vi "Logger.FindData2.vi"() -> ()   [LabVIEW 2016]
uses:
  Logger.File.Serials.ctl
  Sequence/Sequence.Step.Status.ctl
panel:
  out "spreadsheet string 2":string
  out "spreadsheet string":string
  out "Array":string[](array[string])
  out "unique values":string[](array[string])
  out "sum":i16
  out "sorted array 2":T1(array[cluster])
  out "Data":T2[][](array[typedef])
  out "error out":errorcluster
  out "size(s)":i32
  in  "Files":path[](array[path])=[path "D:/Maszup/WABCO/SVN/LaserMarkingStation/SOFTWARE/logs/results1/new/170424160700 899 053 814 4.tdms", path "D:/Maszup/WABCO/SVN/LaserMarkingStation/SOFTWARE/logs/results1/new/170425142313 899 053 814 4.tdms", path "D:/Maszup/WABCO/SVN/LaserMarkingStation/SOFTWARE/logs/results1/new/170425154602 899 053 814 4.tdms", path "D:/Maszup/WABCO/SVN/LaserMarkingStation/SOFTWARE/logs/results1/new/170425215851 899 053 814 4.tdms", path "D:/Maszup/WABCO/SVN/LaserMarkingStation/SOFTWARE/logs/results1/new/170427101020 899 053 814 4.tdms", path "D:/Maszup/WABCO/SVN/LaserMarkingStation/SOFTWARE/logs/results1/new/170427132145 899 053 814 4.tdms", path "D:/Maszup/WABCO/SVN/LaserMarkingStation/SOFTWARE/logs/results1/new/170427164857 899 053 814 4.tdms", path "D:/Maszup/WABCO/SVN/LaserMarkingStation/SOFTWARE/logs/results1/old/170404114910 899 053 814 4.tdms", path "D:/Maszup/WABCO/SVN/LaserMarkingStation/SOFTWARE/logs/results1/old/170404165439 899 053 814 4.tdms", path "D:/Maszup/WABCO/SVN/LaserMarkingStation/SOFTWARE/logs/results1/old/170404212337 899 053 814 4.tdms", path "D:/Maszup/WABCO/SVN/LaserMarkingStation/SOFTWARE/logs/results1/old/170406132445 899 053 814 4.tdms", path "D:/Maszup/WABCO/SVN/LaserMarkingStation/SOFTWARE/logs/results1/old/170406155100 899 053 814 4.tdms", path "D:/Maszup/WABCO/SVN/LaserMarkingStation/SOFTWARE/logs/results1/old/170406203614 899 053 814 4.tdms", path "D:/Maszup/WABCO/SVN/LaserMarkingStation/SOFTWARE/logs/results1/old/170408024126 899 053 814 4.tdms", path "D:/Maszup/WABCO/SVN/LaserMarkingStation/SOFTWARE/logs/results1/old/170408025114 899 053 814 4.tdms", path "D:/Maszup/WABCO/SVN/LaserMarkingStation/SOFTWARE/logs/results1/old/170408033252 899 053 814 4.tdms", path "D:/Maszup/WABCO/SVN/LaserMarkingStation/SOFTWARE/logs/results1/old/170410070739 899 053 814 4.tdms", path "D:/Maszup/WABCO/SVN/LaserMarkingStation/SOFTWARE/logs/results1/old/170410115154 899 053 814 4.tdms", path "D:/Maszup/WABCO/SVN/LaserMarkingStation/SOFTWARE/logs/results1/old/170411223457 899 053 814 4.tdms", path "D:/Maszup/WABCO/SVN/LaserMarkingStation/SOFTWARE/logs/results1/old/170412013424 899 053 814 4.tdms", path "D:/Maszup/WABCO/SVN/LaserMarkingStation/SOFTWARE/logs/results1/old/170412052729 899 053 814 4.tdms", path "D:/Maszup/WABCO/SVN/LaserMarkingStation/SOFTWARE/logs/results1/old/170413051815 899 053 814 4.tdms", path "D:/Maszup/WABCO/SVN/LaserMarkingStation/SOFTWARE/logs/results1/old/170413111535 899 053 814 4.tdms", path "D:/Maszup/WABCO/SVN/LaserMarkingStation/SOFTWARE/logs/results1/old/170413172133 899 053 814 4.tdms", path "D:/Maszup/WABCO/SVN/LaserMarkingStation/SOFTWARE/logs/results1/old/170414192304 899 053 814 4.tdms", path "D:/Maszup/WABCO/SVN/LaserMarkingStation/SOFTWARE/logs/results1/old/170419031847 899 053 814 4.tdms", path "D:/Maszup/WABCO/SVN/LaserMarkingStation/SOFTWARE/logs/results1/old/170419071455 899 053 814 4.tdms", path "D:/Maszup/WABCO/SVN/LaserMarkingStation/SOFTWARE/logs/results2/new/170420162556 899 053 814 4.tdms", path "D:/Maszup/WABCO/SVN/LaserMarkingStation/SOFTWARE/logs/results2/new/170421075116 899 053 814 4.tdms", path "D:/Maszup/WABCO/SVN/LaserMarkingStation/SOFTWARE/logs/results2/new/170424124919 899 053 814 4.tdms", path "D:/Maszup/WABCO/SVN/LaserMarkingStation/SOFTWARE/logs/results2/new/170425130831 899 053 814 4.tdms"]
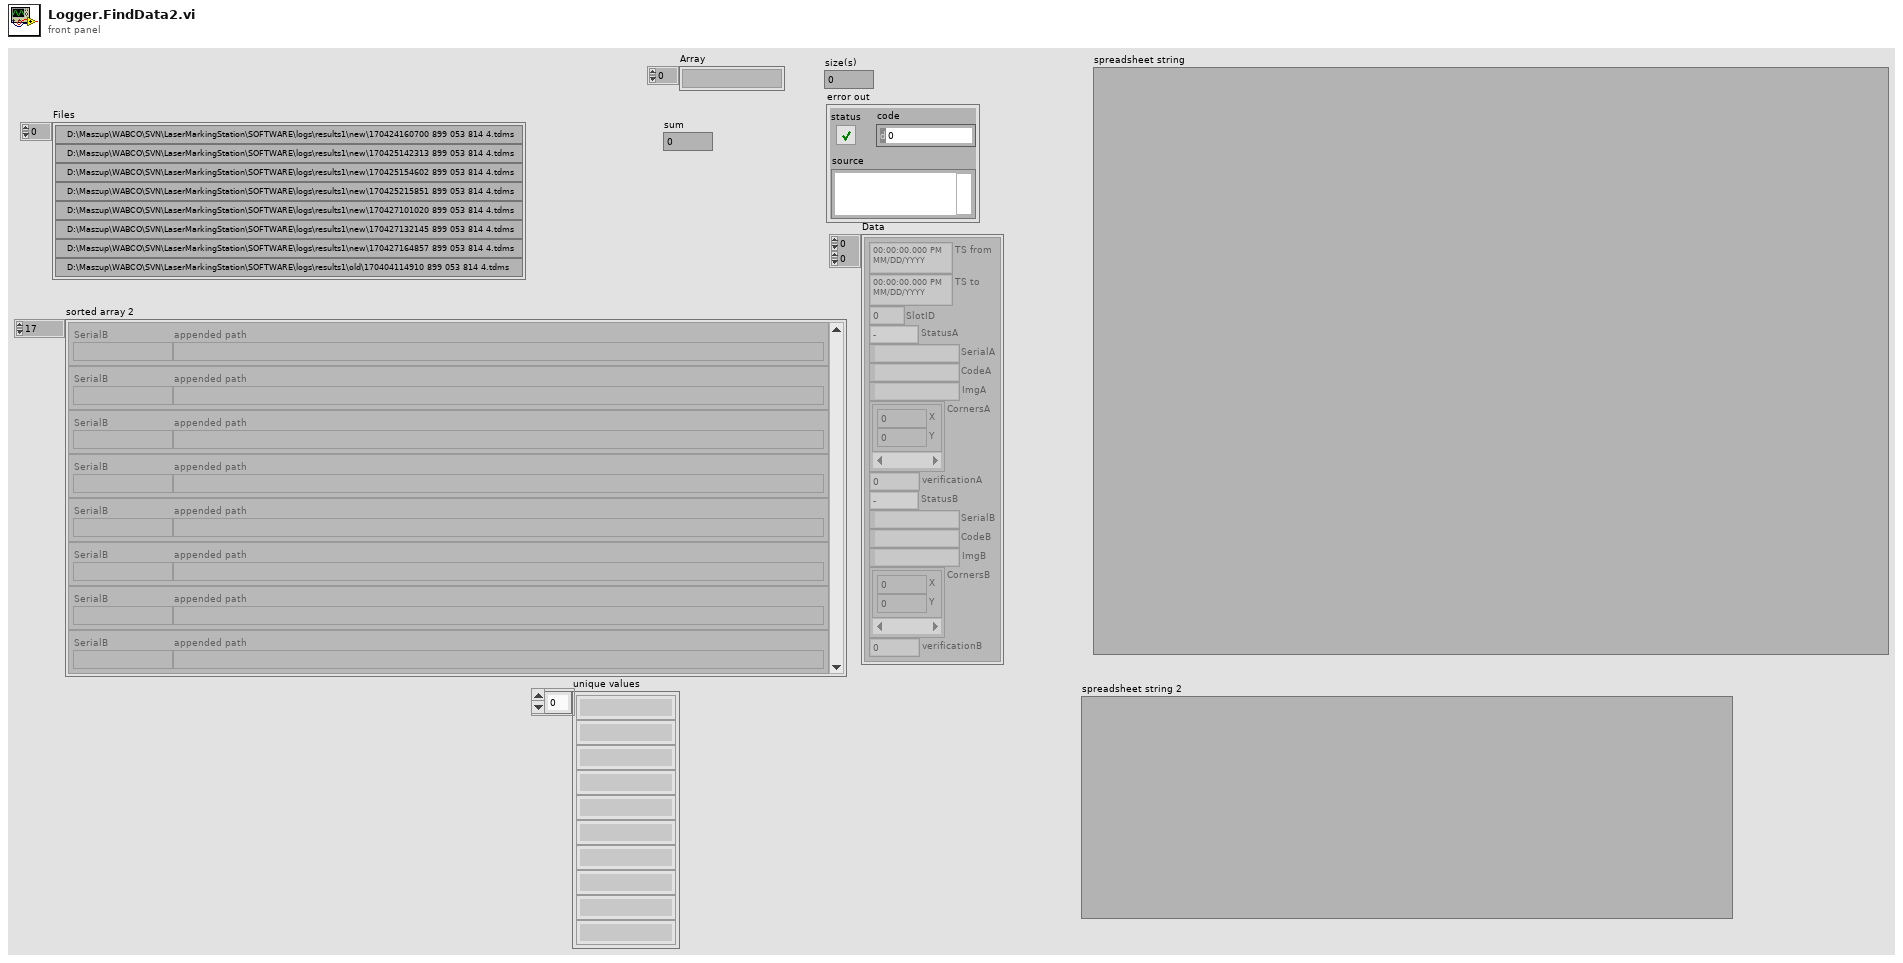
[diagram p1: front panel]
types:
  T1 = cluster{"SerialB":string, "appended path":path}[]
  T2 = typedef "Logger.File.Serials.ctl" = cluster{"TS from":timestamp, "TS to":timestamp, "SlotID":u8, "StatusA":T3, "SerialA":string, "CodeA":string, "ImgA":string, "CornersA":cluster{"X":i32, "Y":i32}[], "verificationA":u8, "StatusB":T3, "SerialB":string, "CodeB":string, "ImgB":string, "CornersB":cluster{"X":i32, "Y":i32}[], "verificationB":u8}
  T3 = typedef "Sequence.Step.Status.ctl" = enum16{"-", "Pending", "Running", "Skipped", "Passed", "Failed", "Done", "Error", "Aborted", "Stopped"}
  T4 = enum16{"open", "open or create", "create or replace", "create", "open (read-only)"}
  T5 = cluster{"SerialB":string, "appended path":path, i32}
  T6 = cluster{"SerialB":string, "appended path":path, i32}[]
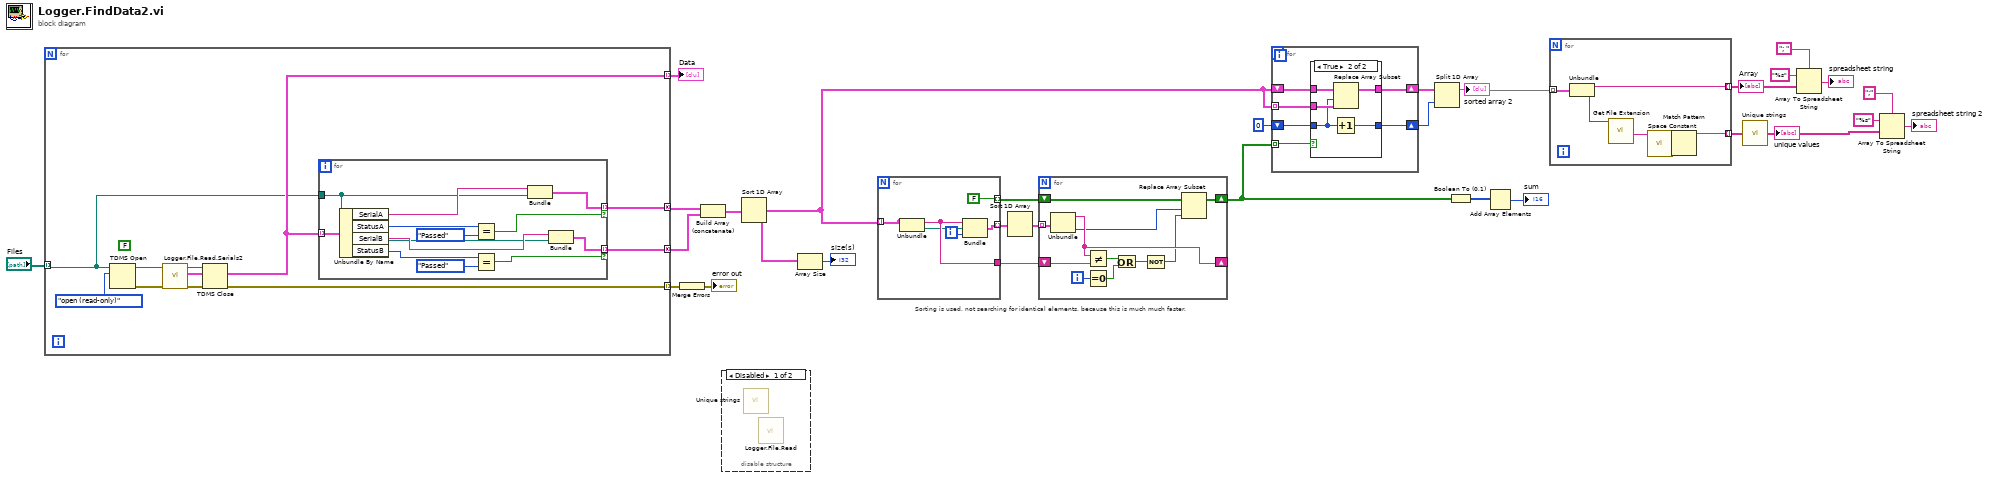
[diagram p0: block diagram]
diagram:
  # "Sorting is used, not searching for identical elements, because this is much much faster."
  n1 = for {
    tunnel: "Files" -> [w30] mode=indexing
    tunnel: [w32] -> w26 mode=indexing
    tunnel: [w39] -> w23 mode=concatenating
    tunnel: [w38] -> w24 mode=concatenating
    tunnel: [w31] -> w22 mode=indexing
    (unwired) FALSE ("create index file? (T)")
    n2 = TDMS Open(10:T4."open (read-only)" ("operation (0:open)"), 11:w30) -> (0:w35:errorcluster, 3:w36:refnum<k34>)  [unwired: 5 in]
    n3 = call "Logger.File.Read.Serials2.vi"("error in"=w35, "file ref in"=w36) -> ("error out"=w34:errorcluster, "Data"=w31:T2[], "file ref out"=w33:refnum<k34>)  [unwired: 7 in]
    n4 = TDMS Close(8:w34, 11:w33) -> (0:w32:errorcluster)  [unwired: 1 out]
    n5 = for {
      tunnel: [w40] -> w39 mode=indexing if=w47
      tunnel: [w41] -> w38 mode=indexing if=w46
      tunnel: w31 -> [w45] mode=indexing
      tunnel: w30 -> [w42]
      n6 = Unbundle By Name(w45) -> ("SerialA"=w44:string, "StatusA"=w51:T3, "SerialB"=w43:string, "StatusB"=w48:T3)
      n7 = Equal?(x=w51, y=Sequence.Step.Status."Passed") -> (x = y?=w46:bool)
      n8 = Equal?(x=w48, y=Sequence.Step.Status."Passed") -> (x = y?=w47:bool)
      n9 = Bundle("SerialA"=w44, "appended path"=w42) -> (w41:cluster{"SerialA":string, "appended path":path})  [unwired: 1 in]
      n10 = Bundle("SerialB"=w43, "appended path"=w42) -> (w40:cluster{"SerialB":string, "appended path":path})  [unwired: 1 in]
    }
  }
  "Data" <- w22
  n11 = Merge Errors(w26) -> (→"error out":errorcluster)
  n12 = Build Array (concatenate)(w24, w23) -> (w28:T1)
  n13 = disable-structure shown="Disabled" {
    frame Disabled {
      n14 = call "Unique strings.vi"() -> ()  [unwired: 1 in, 1 out]
      n15 = call "Logger.File.Read.vi"() -> ()  [unwired: 8 in, 4 out]
    }
    frame Enabled {
    }
  }
  n16 = Sort 1D Array(array=w28) -> (sorted array=w12:T1)
  n17 = Array Size(array=w12) -> (size(s)=→"size(s)":i32)
  n18 = for {
    tunnel: [w54] -> _ mode=indexing
    tunnel: [w56] -> w21 mode=indexing
    tunnel: [FALSE] -> w18 mode=indexing
    tunnel: [w53] -> w20
    tunnel: w12 -> [w54] mode=indexing
    i -> [w57]
    n19 = Unbundle(w54) -> ("SerialB"=w53:string, "appended path"=w52:path)
    n20 = Bundle("SerialB"=w53, "appended path"=w52, w57) -> (w56:T5)  [unwired: 1 in]
  }
  n21 = Sort 1D Array(array=w21) -> (sorted array=w19:T6)
  n22 = for {
    shift-right: [w61] -> _
    shift-left: w20 -> [w62]
    tunnel: w19 -> [w68] mode=indexing
    shift-right: [w66] -> w11
    shift-left: w18 -> [w67]
    i -> [w65]
    n23 = Unbundle(w68) -> ("SerialB"=w61:string, w59:i32)  [unwired: 1 out]
    n24 = Not Equal?(x=w61, y=w62) -> (x != y?=w63:bool)
    n25 = Equal To 0?(x=w65) -> (x = 0?=w64:bool)
    n26 = Or(x=w63, y=w64) -> (x .or. y?=w60:bool)
    n27 = Not(x=w60) -> (.not. x?=w58:bool)
    n28 = Replace Array Subset(array=w67, new element=w58, index=w59) -> (w66:bool[])
  }
  n29 = for {
    tunnel: w11 -> [w74] mode=indexing
    tunnel: w12 -> [w71] mode=indexing
    shift-right: [w72] -> w14
    shift-left: w12 -> [w73]
    shift-right: [w69] -> w13
    shift-left: 0 -> [w70]
    n30 = case shown="True" w74 {
      tunnel: w73 -> [w76 w81]
      tunnel: [w76 w80] -> w72
      tunnel: w71 -> [_ w79]
      tunnel: w70 -> [w75 w78]
      tunnel: [w75 w77] -> w69
      frame False {
      }
      frame True {
        n31 = Replace Array Subset(array=w81, new element=w79, index=w78) -> (w80:T1)
        n32 = Increment(x=w78) -> (x+1=w77:i32)
      }
    }
  }
  n33 = Split 1D Array(array=w14, index=w13) -> (first subarray=w10:T1)  [unwired: 1 out]
  "sorted array 2" <- w10
  n34 = Boolean To (0,1)(Boolean=w11) -> (0, 1=w17:i16[])
  n35 = Add Array Elements(numeric array=w17) -> (sum=→"sum":i16)
  n36 = for {
    tunnel: w10 -> [w87] mode=indexing
    tunnel: [w86] -> w8 mode=indexing
    tunnel: [w83] -> w9 mode=indexing
    n37 = Unbundle(w87) -> ("SerialB"=w86:string, "appended path"=w85:path)
    n38 = call <vilib>:"Get File Extension.vi"("file"=w85) -> ("filename without extension"=w84:string)  [unwired: 6 in, 4 out]
    n39 = call <vilib>:"Space Constant.vi"() -> ("String"=w82:string)
    n40 = Match Pattern(string=w84, regular expression=w82) -> (before substring=w83:string)  [unwired: 1 in, 3 out]
  }
  "Array" <- w8
  n41 = call "Unique strings.vi"("values in"=w9) -> ("unique values"=w2:string[])
  "unique values" <- w2
  n42 = Array To Spreadsheet String(delimiter (Tab)="; ", array=w8, 3:"%s" ("format string")) -> (spreadsheet string=→"spreadsheet string":string)
  n43 = Array To Spreadsheet String(delimiter (Tab)=";", array=w2, 3:"%s" ("format string")) -> (spreadsheet string=→"spreadsheet string 2":string)
